vi "Get FirstPopulatedQueue.vi"(8 "error in":errorcluster, 10 "Timeout (-1 ms)":i32=-1, 11 "PriorityMessageQueue in":refnum<class "PriorityMessageQueue.lvclass">) -> (0 "error out":errorcluster, 2 "MsgQ":refnum<queue>, 3 "PriorityMessageQueue out":refnum<class "PriorityMessageQueue.lvclass">, 4 "Timeout":bool)   [LabVIEW 2009, in "LapDog.Messaging.v2.lvlib" / "PriorityMessageQueue.lvclass"]
uses:
  PriorityMessageQueue.lvclass
  MessageObject/Message.lvclass
  PriorityMessageQueue.lvclass/PriorityMessageQueue.ctl
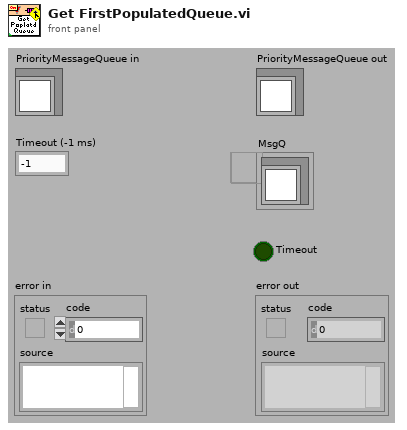
[diagram p1: front panel]
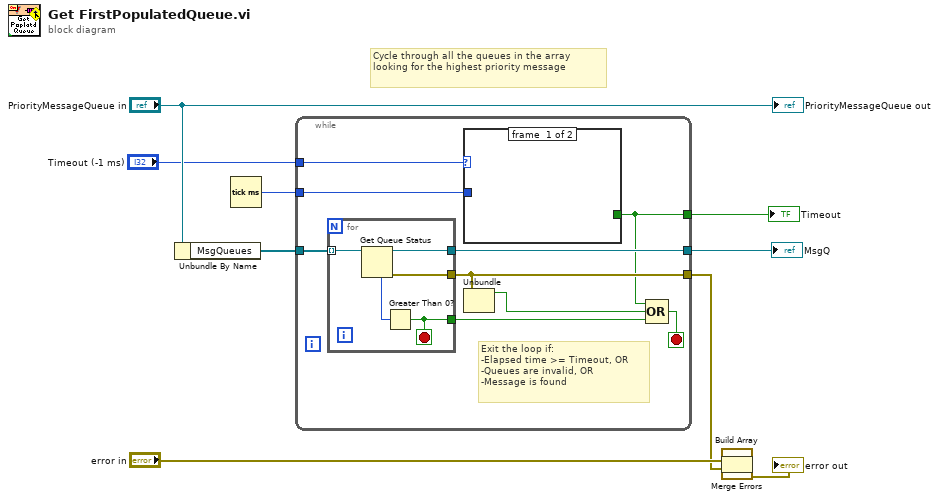
[diagram p0: block diagram]
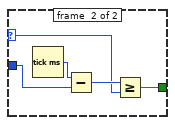
[diagram p2: hidden frame]
diagram:
  # "Cycle through all the queues in the array looking for the highest priority message"
  n1 = Unbundle By Name("PriorityMessageQueue in") -> ("MsgQueues"=w9:refnum<queue>[])
  n2 = Tick Count (ms)() -> (millisecond timer value=w3:u32)
  n3 = while {
    tunnel: w9 -> [w19]
    tunnel: [w18] -> w8
    tunnel: [w16] -> w6
    tunnel: "Timeout (-1 ms)" -> [w12]
    tunnel: w3 -> [w13]
    tunnel: [w11] -> w2
    stop <- w15 stop-if-true
    # "Exit the loop if:\n-Elapsed time >= Timeout, OR\n-Queues are invalid, OR\n-Message is found"
    n4 = for {
      tunnel: w19 -> [w29] mode=indexing
      tunnel: [w27] -> w18
      tunnel: [w26] -> w16
      tunnel: [w25] -> w17
      stop <- w25 stop-if-true
      n5 = Get Queue Status(queue=w29) -> (queue out=w27:refnum<queue>, error out=w26:errorcluster, # elements in queue=w28:i32)  [unwired: 2 in, 5 out]
      n6 = Greater Than 0?(x=w28) -> (x > 0?=w25:bool)
    }
    n7 = case shown="0.." w12 {
      selector: w12 -> [_ w21]
      tunnel: w13 -> [_ w24]
      tunnel: [_ w20] -> w11
      frame #0 {
      }
      frame #1 {
        n8 = Tick Count (ms)() -> (millisecond timer value=w23:u32)
        n9 = Subtract(x=w23, y=w24) -> (x-y=w22:u32)
        n10 = Greater Or Equal?(x=w22, y=w21) -> (x >= y?=w20:bool)
      }
    }
    n11 = Unbundle(w16) -> ("status"=w14:bool)  [unwired: 2 out]
    n12 = Compound Arithmetic op=OR(w11, w14, w17) -> (w15:bool)
  }
  "MsgQ" <- w8
  "Timeout" <- w2
  n13 = Build Array("error in", w6) -> (w1:errorcluster[])
  n14 = call <vilib>:"Merge Errors.vi"("error array in"=w1) -> ("error out"=→"error out":errorcluster)  [unwired: 6 in]
  "PriorityMessageQueue out" <- "PriorityMessageQueue in"
